vi "Pre Launch Init.vi"(11 "Logger in":refnum<class "Generic Logger.lvclass">) -> (0 "error out":errorcluster, 3 "Logger out":refnum<class "Generic Logger.lvclass">)   [LabVIEW 2020, in "Logging.lvlib" / "Generic Logger.lvclass"]
doc: "(<B>Filename</B>: Actor Framework.lvlib:Actor.lvclass:Pre Launch Init.vi)\n\nDefines behavior that occurs after the Launch Nested Actor method is invoked but before the actor's Actor Core method begins running.\n\nBy default, this method does nothing. A descendant class may override it to define behavior."
uses:
  Generic Logger.lvclass
  Generic Logger.lvclass/Generic Logger.ctl
  <vilib>/ActorFramework/Actor/Actor.lvclass
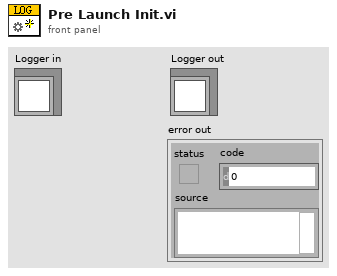
[diagram p1: front panel]
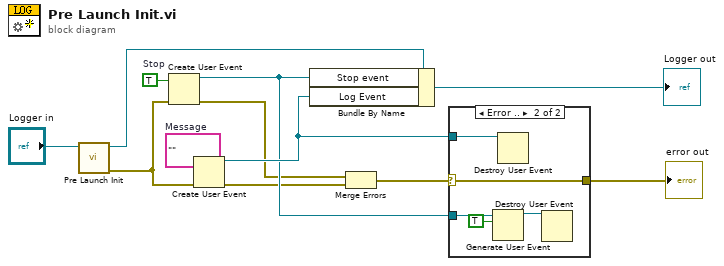
[diagram p0: block diagram]
diagram:
  w6 = TRUE  # Stop
  w11 = ""  # Message
  n1 = call-parent "Pre Launch Init.vi"("Actor in"="Logger in") -> ("error out"=w1:errorcluster, "Actor out"=w9:refnum<class "Generic Logger.lvclass">)  [unwired: 9 in]
  n2 = Create User Event(user event datatype=w6, error in=w1) -> (user event=w5:refnum<user-event>, error out=w4:errorcluster)
  n3 = Create User Event(user event datatype=w11, error in=w1) -> (user event=w10:refnum<user-event>, error out=w3:errorcluster)
  n4 = Bundle By Name(cluster=w9, "Stop event"=w5, "Log Event"=w10) -> (→"Logger out":refnum<class "Generic Logger.lvclass">)
  n5 = Merge Errors(w4, w3) -> (w2:errorcluster)
  n6 = case shown="Error .." w2 {
    selector: w2 -> [w13 w17]
    tunnel: w10 -> [_ w18]
    tunnel: [w13 w17] -> w7
    tunnel: w5 -> [_ w16]
    frame No Error {
    }
    frame Error {
      n7 = Generate User Event(user event=w16, event data cluster=TRUE ("event data")) -> (user event out=w15:refnum<user-event>)  [unwired: 2 in, 1 out]
      n8 = Destroy User Event(user event=w18) -> ()  [unwired: 1 in, 1 out]
      n9 = Destroy User Event(user event=w15) -> ()  [unwired: 1 in, 1 out]
    }
  }
  "error out" <- w7
